vi "Get SMO Serial Number.vi"(8 "error in (no error)":errorcluster, 11 "Instrument.AFM_DLog in":refnum<class "Instrument.AFM_DLog.lvclass">) -> (0 "error out":errorcluster, 2 "Serial Number":string, 3 "Instrument.AFM_DLog out":refnum<class "Instrument.AFM_DLog.lvclass">)   [LabVIEW 2019, in "Instrument.AFM_DLog.lvclass"]
doc: "Override this VI to return the port number of your Instrument"
uses:
  Instrument.AFM_DLog.lvclass
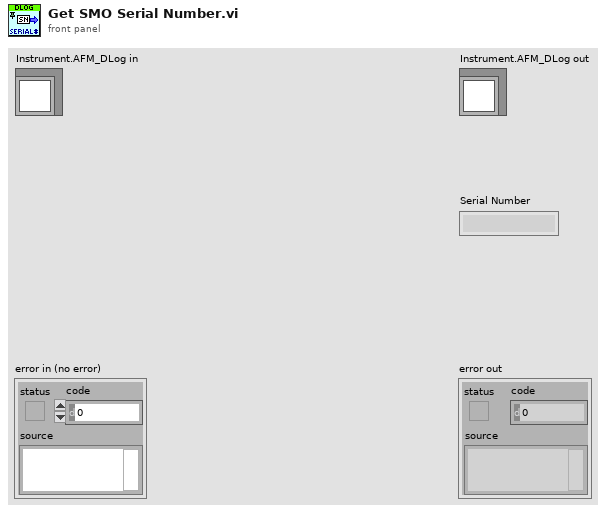
[diagram p1: front panel]
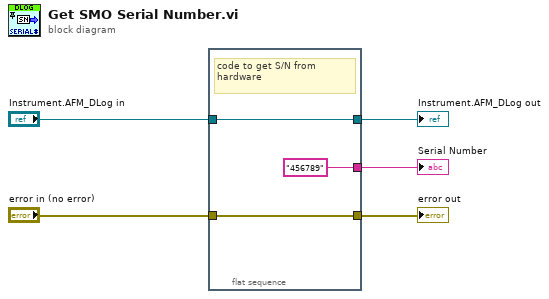
[diagram p0: block diagram]
diagram:
  n1 = flat-sequence {
    tunnel: "Instrument.AFM_DLog in" -> [w8]
    tunnel: [w8] -> w4
    tunnel: [w7] -> w3
    tunnel: "error in (no error)" -> [w7]
    tunnel: ["456789" ("Serial Number")] -> w1
    frame #0 {
      # "code to get S/N from hardware"
    }
  }
  "error out" <- w3
  "Instrument.AFM_DLog out" <- w4
  "Serial Number" <- w1
